vi "Configure AC Line Trigger Slope.vi"(8 "error in (no error)":errorcluster {"code" format="%.0x"}, 10 "AC Line Slope (Positive)":i32(slide), 11 "VISA Resource Name":refnum<visa-resource-name>) -> (0 "error out":errorcluster {"code" format="%.0x"}, 3 "VISA Resource Name Out":refnum<visa-resource-name>)   [LabVIEW 2010, in "Tektronix TDS 3000 Series.lvlib"]
doc: "This VI configures the oscilloscope for AC Line triggering.\n\nNotes:\n\n(1) This VI affects instrument behavior only if the Trigger Type is AC Line Trigger. Call the Configure Trigger VI to set the Trigger Type before you call this VI."
uses:
  <instrlib>/Tektronix TDS 3000 Series/Tektronix TDS 3000 Series.lvlib
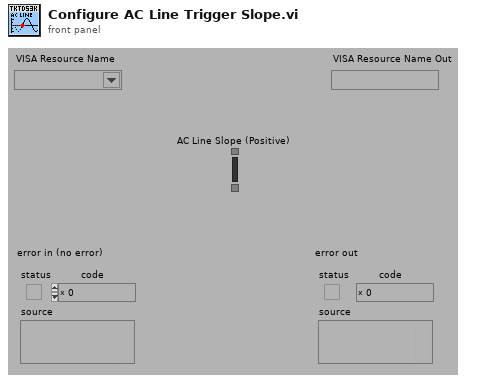
[diagram p1: front panel]
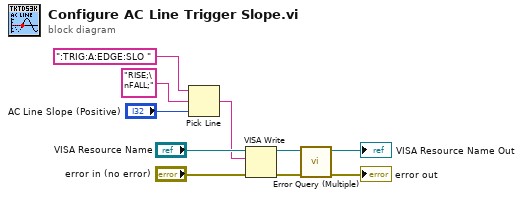
[diagram p0: block diagram]
diagram:
  n1 = Pick Line(string ("")=":TRIG:A:EDGE:SLO ", multi-line string="RISE;\nFALL;", line index="AC Line Slope (Positive)") -> (output string=w6:string)
  n2 = VISA Write(VISA resource name="VISA Resource Name", write buffer=w6, error in (no error)="error in (no error)") -> (VISA resource name out=w4:refnum<visa-resource-name>, error out=w3:errorcluster)  [unwired: 1 out]
  n3 = call <instrlib>:"Error Query (Multiple).vi"("error in (no error)"=w3, "VISA Resource Name"=w4) -> ("error out"=→"error out":errorcluster, "VISA Resource Name Out"=→"VISA Resource Name Out":refnum<visa-resource-name>)  [unwired: 6 in, 2 out]
